vi "Get Serial Interface Max Baud.vi"(8 "Error In":errorcluster, 11 "LINX Device Config":T1) -> (0 "Error Out":errorcluster, 2 "Baud Rate":u32, 3 "LINX Device Config":T1)   [LabVIEW 2011, in "LVH-LINX.lvlib" / "Device.lvlib"]
doc: "Get the maximum baud rate the LINX device is capable of using to communicate with the host."
uses:
  Device.lvlib
  Type Defs/LINX Device Config.ctl
  Type Defs/Interface.ctl
  Type Defs/TCP Config.ctl
  Type Defs/Channels.ctl
  Type Defs/Error Type.ctl
  LVH-LINX.lvlib
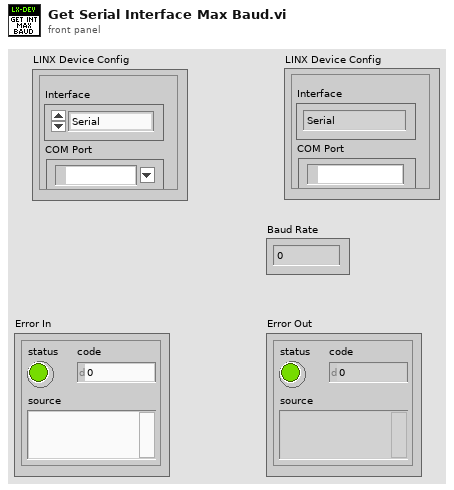
[diagram p1: front panel]
types:
  T1 = typedef "LVH-LINX.lvlib/Device.lvlib/LINX Device Config.ctl" = cluster{"Interface":T2, "COM Port":refnum<visa-resource-name>, "TCP Configuration":T3, "Device Family":u8, "Device ID":u8, "Device Name":string, "TCP Ref":refnum<k5>, "Channels":T4}
  T2 = typedef "LVH-LINX.lvlib/Interface.ctl" = enum16{"Serial", "TCP"}
  T3 = typedef "LVH-LINX.lvlib/Device.lvlib/TCP Config.ctl" = cluster{"IP Address":string, "Port":u16}
  T4 = typedef "LVH-LINX.lvlib/Channels.ctl" = cluster{"DI Channels":u8[], "DO Channels":u8[], "AI":u8[], "AO":u8[], "PWM":u8[], "QE":u8[], "UART":u8[], "I2C 2":u8[], "SPI":u8[], "CAN":u8[], "AI Ref (V)":dbl, "AO Resolution (Bits)":u8, "AO Ref (V)":dbl}
  T5 = typedef "LVH-LINX.lvlib/Error Type.ctl" = enum16{"Unknown", "Timeout", "Corrupt Return Packet", "Unable To Connect", "Command Not Supported", "Channel DNE", "Invalid COM Config", "Firmware Version Mismatch", "myRIO Support"}
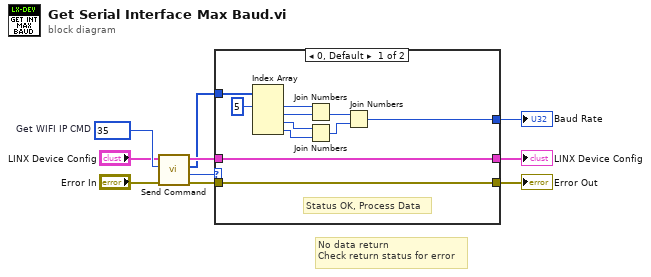
[diagram p0: block diagram]
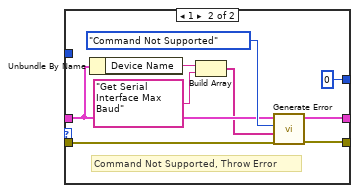
[diagram p2: hidden frame]
diagram:
  w9 = u16 35  # Get WIFI IP CMD
  # "No data return\nCheck return status for error"
  n1 = call "Send Command.vi"("Error In"="Error In", "CMD"=w9, "LINX Device Config"="LINX Device Config") -> ("Error Out"=w4:errorcluster, "Status"=w2:u8, "Response"=w3:u8[], "LINX Device Config"=w6:T1)  [unwired: 5 in]
  n2 = case shown="0, Default" w2 {
    tunnel: [w20 w28] -> w7
    tunnel: w6 -> [w20 w24]
    tunnel: [w21 w29] -> w5
    tunnel: w4 -> [w21 w30]
    tunnel: w3 -> [w19 _]
    tunnel: [w15 u32 0] -> w1
    frame 0, Default {
      # "Status OK, Process Data"
      n3 = Index Array(array=w19, index #1=5 ("index")) -> (element #1=w17:u8, element #2=w16:u8, element #3=w12:u8, element #4=w11:u8)  [unwired: 3 in]
      n4 = Join Numbers(hi=w17, lo=w16) -> ((hi.lo)=w14:u16)
      n5 = Join Numbers(hi=w12, lo=w11) -> ((hi.lo)=w13:u16)
      n6 = Join Numbers(hi=w14, lo=w13) -> ((hi.lo)=w15:u32)
    }
    frame 1 {
      # "Command Not Supported, Throw Error"
      n7 = Unbundle By Name(w24) -> ("Device Name"=w25:string)
      n8 = Build Array(w25, "Get Serial Interface Max Baud") -> (w23:string[])
      n9 = call "Generate Error.vi"("Error In"=w30, "Arguments"=w23, "Error Type"=Error_Type."Command Not Supported", "LINX Device Config"=w24) -> ("Error Out"=w29:errorcluster, "LINX Device Config"=w28:T1)  [unwired: 6 in]
    }
  }
  "Error Out" <- w5
  "LINX Device Config" <- w7
  "Baud Rate" <- w1
